vi "Convertir_Opcion(SubVI).vi"(9 "Figura Geometrica X":T1, 10 "Eje de la Figura X":T2, 11 "Operación X":T3) -> (3 "Numeric Control":i32)   [LabVIEW 2017]
uses:
  Control_Operacion.ctl
  Control_Eje_Figura.ctl
  Control_Figura.ctl
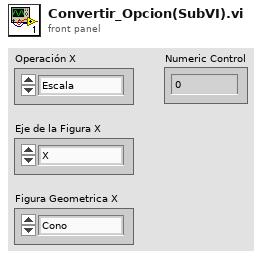
[diagram p1: front panel]
types:
  T1 = typedef "Control_Figura.ctl" = enum16{"Cono", "Esfera", "Cilindro"}
  T2 = typedef "Control_Eje_Figura.ctl" = enum16{"X", "Y", "Z"}
  T3 = typedef "Control_Operacion.ctl" = enum16{"Escala", "Translación", "Rotación"}
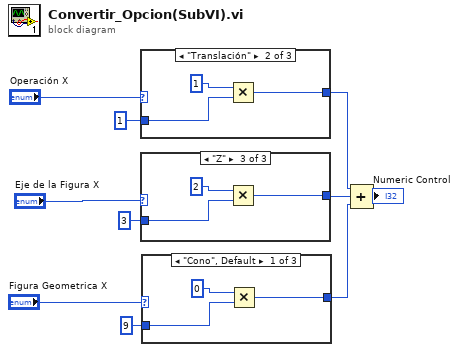
[diagram p0: block diagram]
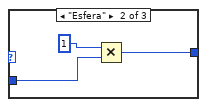
[diagram p2: hidden frame]
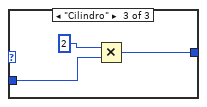
[diagram p3: hidden frame]
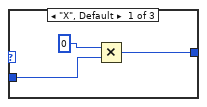
[diagram p4: hidden frame]
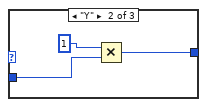
[diagram p5: hidden frame]
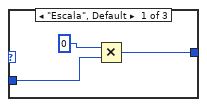
[diagram p6: hidden frame]
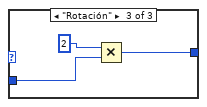
[diagram p7: hidden frame]
diagram:
  n1 = case shown="\"Translación\"" "Operación X" {
    tunnel: [w12 w15 w18] -> w6
    tunnel: 1 ("y") -> [w11 w14 w17]
    frame "Escala", Default {
      n2 = Multiply(x=0, y=w11) -> (x*y=w12:i32)
    }
    frame "Translación" {
      n3 = Multiply(x=1, y=w14) -> (x*y=w15:i32)
    }
    frame "Rotación" {
      n4 = Multiply(x=2, y=w17) -> (x*y=w18:i32)
    }
  }
  n5 = case shown="\"Z\"" "Eje de la Figura X" {
    tunnel: [w21 w24 w27] -> w4
    tunnel: 3 ("y") -> [w20 w23 w26]
    frame "X", Default {
      n6 = Multiply(x=0, y=w20) -> (x*y=w21:i32)
    }
    frame "Y" {
      n7 = Multiply(x=1, y=w23) -> (x*y=w24:i32)
    }
    frame "Z" {
      n8 = Multiply(x=2, y=w26) -> (x*y=w27:i32)
    }
  }
  n9 = case shown="\"Cono\", Default" "Figura Geometrica X" {
    tunnel: [w30 w33 w36] -> w5
    tunnel: 9 ("y") -> [w29 w32 w35]
    frame "Cono", Default {
      n10 = Multiply(x=0, y=w29) -> (x*y=w30:i32)
    }
    frame "Esfera" {
      n11 = Multiply(x=1, y=w32) -> (x*y=w33:i32)
    }
    frame "Cilindro" {
      n12 = Multiply(x=2, y=w35) -> (x*y=w36:i32)
    }
  }
  n13 = Compound Arithmetic op=ADD(w6, w4, w5) -> (→"Numeric Control":i32)
